vi "Simple-Network-Streams-Target.vi"() -> ()   [LabVIEW 2015]
doc: "Demonstrates how to use Network Streams to pass data and commands between two running VIs. This VI passes data to the host VI, based on the frequency specified by the host VI."
uses:
  Program Files (x86)/National Instruments/LabVIEW 2015/examples/Data Communication/Network Streams/Simple Network Streams/support/Network Stream Command.ctl
  <vilib>/userdefined/High Color/nirio_resource_hc.ctl
  Program Files (x86)/National Instruments/LabVIEW 2015/examples/Data Communication/Network Streams/Simple Network Streams/support/Network Stream Global Stop.vi
  <vilib>/FPGAPlugInAG/cRIO-9082/niLvFpga_Open_cRIO-9082.vi
  <vilib>/rvi/interface/common/dynamic/niFpgaDynamicAddResources.vi
  <vilib>/FPGAPlugInAG/Dynamic/niLvFpga_Reset_Dynamic.vi
  <vilib>/rvi/interface/common/niFpgaWaitOnOcc.vi
  <vilib>/Utility/error.llb/Error Cluster From Error Code.vi
  <vilib>/FPGAPlugInAG/Dynamic/niLvFpga_Run_Dynamic.vi
  <vilib>/rvi/errors/niLvFpgaAdjustHostInterfaceError.vi
  <vilib>/ErrorRing/Error Ring.xnode
  <vilib>/rvi/interface/nirviOpenFPGA/nirviOpenFPGA.xnode
  FPGA Bitfiles/afmimagingcontro_FPGATargetSPARTA_raster-scanning_DXF4O8EAjZ4.lvbitx
  <vilib>/rvi/interface/nirviMethod/nirviMethod.xnode
  <resource>/objmgr/ni.dex.rc
  <vilib>/FPGAPlugInAG/Dynamic/niLvFpga_ConfigureFifo_Dynamic.vi
  <vilib>/rvi/errors/niLvFpgaMergeErrorWithErrorCode.vi
  <vilib>/FPGAPlugInAG/Dynamic/niLvFpga_ReadFifo_Dynamic.vi
panel:
  out "Available Elements to Write":i32
  in  "Write Speed":u16(ring)=1 items=["Fast (10 ms)", "Slow (20 ms)"]
  out "Frequency":dbl(knob) scale=10.0..100.0
  in  "Stop":bool
  # "Overview: Demonstrates how to use Network Streams to pass data and commands between two running VIs.\nRequirements: Windows\nInstructions:\n1. Run this VI.\n2. Open Simple Network Streams - Host.vi and follow the instructions on its front panel."
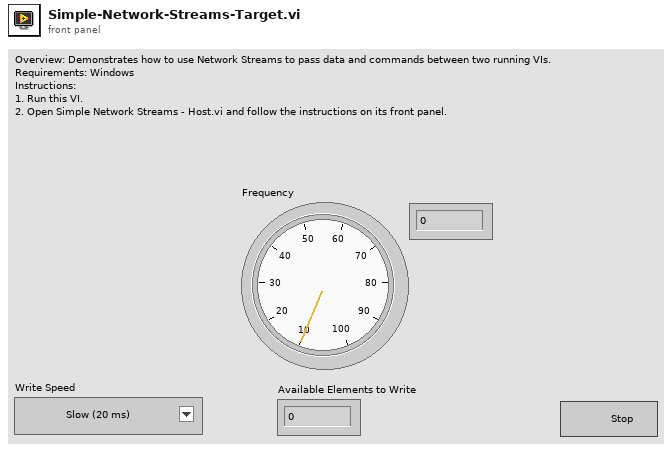
[diagram p1: front panel]
types:
  T1 = typedef "nirio_resource_hc.ctl" = tag
  T2 = typedef "Network Stream Command.ctl" = cluster{"Message":string, "Message Data":variant}
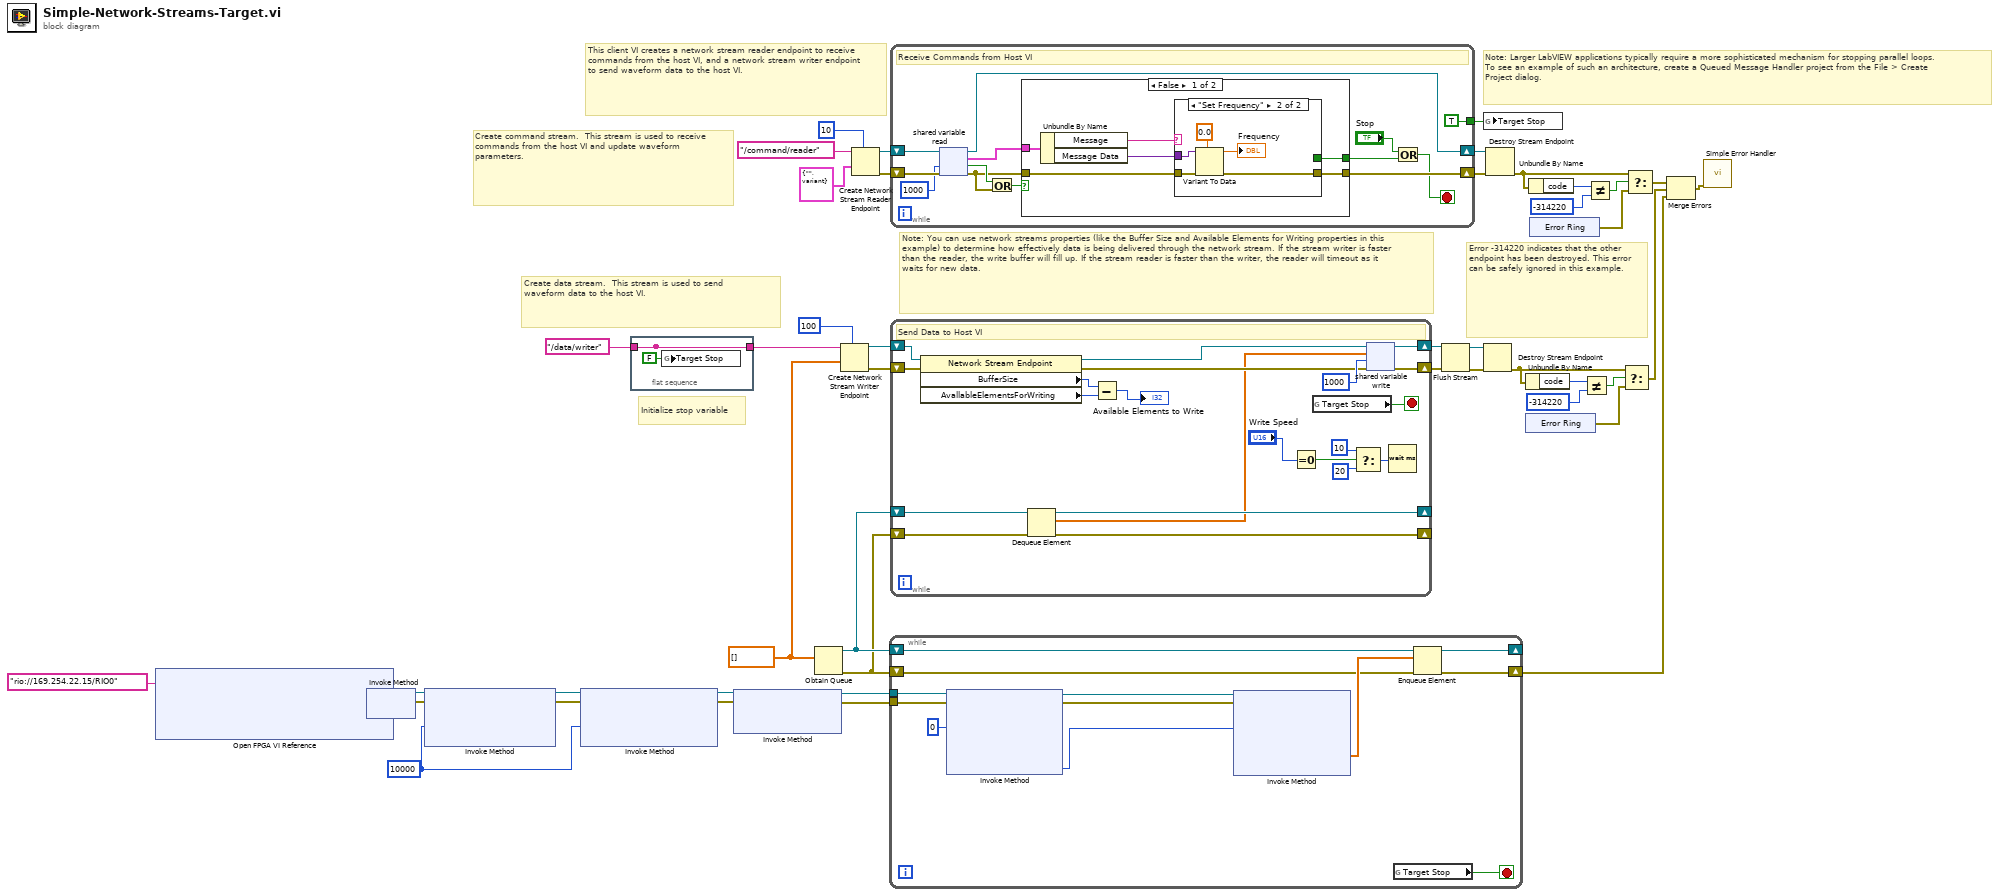
[diagram p0: block diagram]
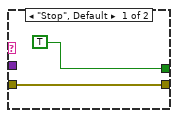
[diagram p2: hidden frame]
diagram:
  w3 = sgl[] []
  w16 = 10000
  # "Initialize stop variable"
  # "This client VI creates a network stream reader endpoint to receive commands from the host VI, and a network stream writer endpoint to send waveform data to the host VI."
  # "Note: You can use network streams properties (like the Buffer Size and Available Elements for Writing properties in this example) to determine how effectively data is being delivered through the network stream. If the stream writer is faster than the reader, the write buffer will fill up. If the stream reader is faster than the writer, the reader will timeout as it waits for new data."
  # "Note: Larger LabVIEW applications typically require a more sophisticated mechanism for stopping parallel loops. To see an example of such an architecture, create a Queued Message Handler project from the File > Create Project dialog."
  # "Error -314220 indicates that the other endpoint has been destroyed. This error can be safely ignored in this example."
  # "Create command stream.  This stream is used to receive commands from the host VI and update waveform parameters."
  # "Create data stream.  This stream is used to send waveform data to the host VI."
  n1 = xnode "Open FPGA VI Reference"("resource name"=T1 "rio://169.254.22.15/RIO0") -> ("FPGA VI Reference Out"=w15:refnum<k20>, "error out"=w14:errorcluster)  [unwired: 1 in]
  n2 = xnode "Invoke Method"("FPGA VI Reference In"=w15, "error in"=w14) -> ("FPGA VI Reference Out"=w10:refnum<k20>, "error out"=w9:errorcluster)
  n3 = xnode "Invoke Method"("FPGA VI Reference In"=w10, "error in"=w9, "Requested Depth"=w16) -> ("FPGA VI Reference Out"=w11:refnum<k20>, "error out"=w12:errorcluster)  [unwired: 1 out]
  n4 = xnode "Invoke Method"("FPGA VI Reference In"=w11, "error in"=w12, "Requested Depth"=w16) -> ("FPGA VI Reference Out"=w8:refnum<k20>, "error out"=w7:errorcluster)  [unwired: 1 out]
  n5 = flat-sequence {
    tunnel: [w47] -> _
    tunnel: [w47] -> w17
    tunnel: "/data/writer" ("reader url") -> [w47]
    frame #0 {
      n6 = global write "Network Stream Global Stop.vi" "Target Stop"(FALSE ("Host Stop")) -> ()
    }
  }
  n7 = xnode "Invoke Method"("FPGA VI Reference In"=w8, "error in"=w7) -> ("FPGA VI Reference Out"=w6:refnum<k20>, "error out"=w5:errorcluster)  [unwired: 1 in]
  n8 = Obtain Queue(element data type=w3) -> (queue out=w2:refnum<queue>, error out=w1:errorcluster)  [unwired: 4 in, 1 out]
  n9 = Create Network Stream Writer Endpoint(7:100 ("writer buffer size"), 9:w3, 11:w17) -> (0:w46:errorcluster, 3:w45:refnum<k21>)  [unwired: 4 in]
  n10 = Create Network Stream Reader Endpoint(7:10 ("reader buffer size"), 9:T2 {"Message"="", "Message Data"=variant} ("Message Cluster"), 11:"/command/reader" ("reader url")) -> (0:w41:errorcluster, 3:w42:refnum<k21>)  [unwired: 4 in]
  n11 = while {
    tunnel: w6 -> [w60]
    tunnel: w5 -> [w59]
    shift-right: [w51] -> w4
    shift-left: w1 -> [w50]
    shift-right: [w53] -> _
    shift-left: w2 -> [w52]
    stop <- w55 stop-if-true
    n12 = xnode "Invoke Method"("FPGA VI Reference In"=w60, "error in"=w59, "Number of Elements"=u32 0) -> ("FPGA VI Reference Out"=w57:refnum<k20>, "error out"=w56:errorcluster, "Elements Remaining"=w49:u32)  [unwired: 1 in, 1 out]
    n13 = xnode "Invoke Method"("FPGA VI Reference In"=w57, "error in"=w56, "Number of Elements"=w49) -> ("Data"=w54:sgl[])  [unwired: 1 in, 3 out]
    n14 = global read "Network Stream Global Stop.vi" "Target Stop"() -> (w55:bool)
    n15 = Enqueue Element(queue=w52, element=w54, error in (no error)=w50) -> (queue out=w53:refnum<queue>, error out=w51:errorcluster)  [unwired: 1 in, 1 out]
  }
  n16 = while "Host->Target Command Reader" {
    shift-right: [w69] -> w40
    shift-left: w41 -> [w73]
    shift-right: [w71] -> w39
    shift-left: w42 -> [w72]
    tunnel: [TRUE] -> w19
    stop <- w65 stop-if-true
    # "Receive Commands from Host VI"
    n17 = shared-variable-read(w72, w73, 1000 ("timeout ms")) -> (w71:refnum<k21>, w62:errorcluster, w64:bool, w67:T2)
    n18 = Or(x=w64, y=w62) -> (x .or. y?=w63:bool)
    n19 = case shown="False" w63 {
      tunnel: w62 -> [w79 w87]
      tunnel: [w78 w87] -> w69
      tunnel: w67 -> [w76 _]
      tunnel: [w77 _] -> w66
      frame False {
        n20 = Unbundle By Name(w76) -> ("Message"=w75:string, "Message Data"=w74:variant)
        n21 = case shown="\"Set Frequency\"" w75 {
          tunnel: w79 -> [w81 w85]
          tunnel: [w81 w84] -> w78
          tunnel: w74 -> [_ w83]
          tunnel: [TRUE _] -> w77
          frame "Stop", Default {
          }
          frame "Set Frequency" {
            n22 = Variant To Data(error in=w85, type=0.0, Variant=w83) -> (data=→"Frequency":dbl, error out=w84:errorcluster)
          }
        }
      }
      frame True {
      }
    }
    n23 = Or(x="Stop", y=w66) -> (x .or. y?=w65:bool)
  }
  n24 = while "Target->Host Data Writer" {
    shift-right: [w99] -> w35
    shift-left: w46 -> [w101]
    shift-right: [w104] -> w44
    shift-left: w45 -> [w103]
    shift-right: [w90] -> _
    shift-left: w2 -> [w92]
    shift-right: [w89] -> _
    shift-left: w1 -> [w91]
    stop <- w98 stop-if-true
    # "Send Data to Host VI"
    n25 = property class="Network Stream Endpoint"(reference=w103, error in=w101) -> (reference out=w102:refnum<k21>, error out=w100:errorcluster, "BufferSize"=w106:i32, "AvallableElementsForWriting"=w107:i32)
    n26 = Dequeue Element(queue=w92, error in (no error)=w91) -> (queue out=w90:refnum<queue>, element=w88:sgl[], error out=w89:errorcluster)  [unwired: 1 in, 1 out]
    n27 = Subtract(x=w106, y=w107) -> (x-y=→"Available Elements to Write":i32)
    n28 = Equal To 0?(x="Write Speed") -> (x = 0?=w94:bool)
    n29 = global read "Network Stream Global Stop.vi" "Target Stop"() -> (w98:bool)
    n30 = Select(t=u32 10 ("milliseconds to wait"), s=w94, f=u32 20 ("milliseconds to wait")) -> (s? t:f=w96:u32)
    n31 = shared-variable-write(w102, w100, w88, 1000 ("timeout ms")) -> (w104:refnum<k21>, w99:errorcluster)  [unwired: 1 out]
    n32 = Wait (ms)(milliseconds to wait=w96) -> ()  [unwired: 1 out]
  }
  n33 = Flush Stream(8:w35, 11:w44) -> (0:w34:errorcluster, 3:w36:refnum<k21>)  [unwired: 2 in, 1 out]
  n34 = global write "Network Stream Global Stop.vi" "Target Stop"(w19) -> ()
  n35 = Destroy Stream Endpoint(8:w34, 11:w36) -> (0:w21:errorcluster)
  n36 = Destroy Stream Endpoint(8:w40, 11:w39) -> (0:w27:errorcluster)
  n37 = Unbundle By Name(w21) -> ("code"=w25:i32)
  n38 = xnode "Error Ring"() -> ("error out"=w22:errorcluster)
  n39 = Unbundle By Name(w27) -> ("code"=w28:i32)
  n40 = xnode "Error Ring"() -> ("error out"=w31:errorcluster)
  n41 = Not Equal?(x=w25, y=-314220) -> (x != y?=w23:bool)
  n42 = Not Equal?(x=w28, y=-314220) -> (x != y?=w30:bool)
  n43 = Select(t=w21, s=w23, f=w22) -> (s? t:f=w20:errorcluster)
  n44 = Select(t=w27, s=w30, f=w31) -> (s? t:f=w26:errorcluster)
  n45 = Merge Errors(w26, w20, w4) -> (w33:errorcluster)
  n46 = call <vilib>:"Simple Error Handler.vi"("error in (no error)"=w33) -> ()  [unwired: 4 in, 5 out]
